vi "LtaGetModuleProperties.vi"(8 "Error In":errorcluster[](array[cluster]), 9 "Event HandlerCall":bool, 10 "arg":string, 11 "Test.lvclass":refnum<class "Test.lvclass">) -> (0 "Error Out":errorcluster[](array[cluster]), 2 "XmlData":string, 3 "Test.lvclass":refnum<class "Test.lvclass">)   [LabVIEW 2018, in "Test.lvclass"]
uses:
  Test.lvclass
  Test.lvclass/Test.ctl
  FGen/MemberClasses/ArbitraryFunction/TypeDefs/Arbs.ctl
  AcPwr/AcPwrPlugins/ChromaAcLoad/TypeDefs/Device(s)Settings.ctl
  AcPwr/AcPwrPlugins/NHRDCPower/TypeDefs/Device(s)Settings.ctl
  AcPwr/AcPwrPlugins/NHRDCPower/TypeDefs/Modules.ctl
  AcPwr/AcPwrPlugins/PacificPowerSource/TypeDefs/Device(s)Settings.ctl
  AcPwr/AcPwrPlugins/NhRegenGridSim/TypeDefs/Device(s)Settings.ctl
  AcPwr/AcPwrPlugins/NhRegenGridSim/TypeDefs/Modules.ctl
  AcPwr/AcPwrPlugins/NHRDCPower/TypeDefs/MeasurementData.ctl
  AcPwr/AcPwrPlugins/ChromaAcLoad/TypeDefs/MeasurementData.ctl
  AcPwr/AcPwrPlugins/ChromaAcLoad/TypeDefs/Measurements.ctl
  AcPwr/AcPwrPlugins/ChromaAcLoad/TypeDefs/MeasurementType.ctl
  Accessors/Read ModuleIDs.vi
  Accessors/Read ErrorSeverity.vi
  <vilib>/Utility/error.llb/Error Cluster From Error Code.vi
  <vilib>/ErrorRing/Error Ring.xnode
  Sync/SyncPlugins/SyncPluginBase/SyncPluginBase.lvclass
  <userlib>/NIST/NISTErrorLib/NISTErrorLib.lvlib
  LV_TestAutomation/Comms_lib/Comms.lvlib
  FGen/FgenPlugins/FgenPluginBaseClass/FgenPluginsBase.lvclass
  Analysis/AnalysisPlugins/AnalysisPluginBaseClass/AnalysisPluginsBase.lvclass
  FGen/MemberClasses/ArbitraryFunction/ArbitraryFunction.lvclass
  AcPwr/AcPwrPlugins/AcPwrBaseClass/AcPwrBase.lvclass
  AcPwr/AcPwrPlugins/ChromaAcLoad/ChromaAcLoad.lvclass
  AcPwr/AcPwrPlugins/PacificPowerSource/PacificPowerSource.lvclass
  AcPwr/AcPwrPlugins/NhRegenGridSim/NHRGridSim.lvclass
  AcPwr/AcPwrPlugins/NHRDCPower/NHRDCPower.lvclass
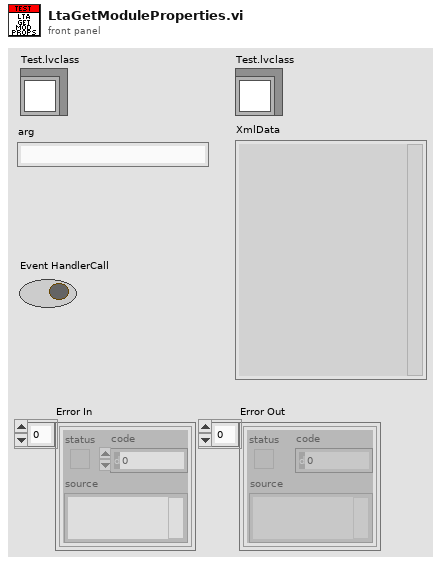
[diagram p1: front panel]
types:
  T1 = typedef "AcPwrPlugins.lvlib/ChromaAcLoad.lvclass/Device(s)Settings.ctl" = cluster{"Configuration Mode":enum16{"Constant Voltage (DC)", "Constant Power (DC)", "Constant Power (AC)", "Constant Current (DC)", "Constant Current (AC)", "Constant Resistance (DC)", "Constant Resistance (AC)", "Rectified Mode (DC)", "Inrush (AC)", "RLC CP (AC)", "RLC (AC)"}, "Phases":cluster{"Handle":string, "Name":string, "Phase Select":i32, "Instrument Options":string, "id query (T)":bool, "reset device (T)":bool, "Load Short Circuited":bool, "Line Synchronization":bool, "Load Current (A/Arms)":dbl, "Load Voltage (V/Vrms)":dbl, "Load Power (W)":dbl, "Load Resistance (Ohms)":dbl, "Load Current Peak Limit (A)":dbl, "Load Current Limit (A/Arms)":dbl, "Load Power Limit (W)":dbl, "Synch Frequency (Hz)":dbl, "Priority":enum16{"CF Only", "PF Only", "Both (CF)", "Both (PF)"}, "Crest Factor":dbl, "Power Factor":dbl, "Slew Rate":cluster{"Rise Slew Rate (A/ms)":i32, "Fall Slew Rate (A/ms)":i32}, "LC/RLC Mode":cluster{"Capacitance (uF)":i32, "Inductance (uH)":i32, "Series Resistance (Ohm)":dbl, "Parallel Resistance (Ohm)":dbl}, "Timing":cluster{"TimingOn":enum16{""}, "Hours":u32, "Minutes":u32, "Seconds":dbl, "CutoffVoltage":dbl}, "Connected":bool}[], "MeasName":string}
  T2 = typedef "AcPwrPlugins.lvlib/PacificPowerSource.lvclass/Device(s)Settings.ctl" = cluster{"MeasName":string, "Modules":cluster{"Handle":string, "Connected":bool, "Clear Device (F)":bool, "btnIdQuery":bool, "btnReset":bool, "Program #":cluster{"Phase B (Degrees)":i32, "Waveform A (1: Sine)":i32, "Voltage Level (Va)":dbl, "Program Number (0)":i32, "Voltage Level (Vb) ":dbl, "Form (3: Three)":u16, "Coupling  (0: Direct)":u16, "Frequency (45Hz)":dbl, "Current Limit (40A)":dbl, "Phase C (Degrees)":i32, "Voltage Level (Vc)":dbl, "Waveform B (1: Sine)":i32, "Waveform C (1: Sine)":i32}[], "Impedance Parameters (off, 0.00)":cluster{"State":bool, "Impedance":dbl}, "Transient Execution (F)":bool, "OutputEnabled":bool, "Source Range":cluster{"Frequency Minimum (45 Hz)":dbl, "Frequency Maximum (1200 Hz)":dbl, "Voltage Maximum (V)":dbl, "Voltage Minimum (V)":dbl, "Range Control (0: Auto)":u16, "Initial Voltage (0V)":u16, "Frequency Range (600Hz)":u16}, "Port Type":enum16{"GPIB", "Serial"}}[]}
  T3 = typedef "AcPwrPlugins.lvlib/NHRGridSim.lvclass/Device(s)Settings.ctl" = cluster{"MeasName":string, "Modules":T4}
  T4 = typedef "AcPwrPlugins.lvlib/NHRGridSim.lvclass/Modules.ctl" = cluster{"Measurement":cluster{"ApertureLength (s)":dbl, "NumberOfSamples":u32}, "Ranges":cluster{"Irange (A)":dbl, "Vrange (V)":dbl}, "Mode":u8, "TransformerRatio":dbl, "Handle":string, "FreqOut (Hz)":dbl, "Connected":bool, "btnIdQuery":bool, "btnReset":bool, "Initialize Timeout ( ms)":u32, "Phase (0: All)":i32, "Grid (0: Normal)":i32, "WatchDog":cluster{"Enable WatchDog":bool, "Robust WatchDog":bool, "Watchdog Interval (s)":dbl}, "Safety Limits":cluster{"Min Voltage (V)":dbl, "Min Voltage Time (s)":dbl, "Max Voltage (V)":dbl, "MaxVoltage Time (s)":dbl, "Max Source Amps (A)":dbl, "Max Source Amps Time (s)":dbl, "Max Sink Amps (A)":dbl, "Max Sink Amps Time (s)":dbl, "Max Source Power (W)":dbl, "Max Source Power Time (s)":dbl, "Max Sink Power (W)":dbl, "Max Sink Power Time (s)":dbl, "Peak Voltage (V)":dbl, "Peak Voltage Enable":bool, "Peak Amps (A)":dbl, "Peak Amps Enable":bool}, "Phases":cluster{"Pout (W)":dbl, "Iout (A)":dbl, "PhaseAngle":dbl, "Vout (V)":dbl, "Phase Name":string}[], "Regulation Gain":dbl, "ChangeOntheFly":bool}[]
  T5 = typedef "AcPwrPlugins.lvlib/ChromaAcLoad.lvclass/MeasurementData.ctl" = cluster{"Time Stamp":timestamp, "Measurements":T6}
  T6 = typedef "AcPwrPlugins.lvlib/ChromaAcLoad.lvclass/Measurements.ctl" = cluster{"Handle":string, "Name":string, "Enabled":bool, "Measurement Value":dbl, "Hold Peak Current Measurement":bool, "btnMeasFetch":bool, "ProtectionStatusString":string, "Measurement Type":T7}[]
  T7 = typedef "AcPwrPlugins.lvlib/ChromaAcLoad.lvclass/MeasurementType.ctl" = enum16{"Voltage (Vrms or V)", "Current (Arms or A)", "Power (W)", "Peak Voltage (V)", "Peak Current (A)", "Peak Power (W)", "Frequency (Hz)", "Resistance (Ohms)", "Voltage Overshoot (V)", "Positive Peak Current (A)", "Voltage Undershoot (V)", "Negative Peak Current (A)", "Apparent Power (VA)", "Reacitive Power (VAR)", "Voltage THD", "Power Factor", "Current's Crest Factor"}
  T8 = typedef "Test.lvclass/SyncEventReg.ctl" = refnum<event-registration>
  T9 = typedef "Test.lvclass/FGenEventReg.ctl" = refnum<event-registration>
  T10 = typedef "Functions.lvlib/ArbitraryFunction.lvclass/Arbs.ctl" = cluster{"Handle":string, "Size":i32, "Gain":dbl, "Offset":dbl}
  T11 = typedef "Test.lvclass/AcPwrEventReg.ctl" = refnum<event-registration>
  T12 = typedef "AcPwrPlugins.lvlib/NHRDCPower.lvclass/Device(s)Settings.ctl" = cluster{"MeasName":string, "Modules":T13}
  T13 = typedef "AcPwrPlugins.lvlib/NHRDCPower.lvclass/Modules.ctl" = cluster{"Handle":string, "Name":string, "id query (Yes)":bool, "reset device (Yes)":bool, "Connected":bool, "Initial Battery Detect Voltage (0)":dbl, "SafetySettings":cluster{"SetWatchDog?":bool, "Voltage (V)":dbl, "Current (A)":dbl, "Power (W)":dbl, "Voltage Delay (s)":dbl, "Current Delay (s)":dbl, "Power Delay (s)":dbl}, "Options String":string, "Aperture Time (s)":dbl, "operating state (Off)":i32, "OutputSettings":cluster{"Voltage (V)":dbl, "Current (A)":dbl, "Resistance (Ohms)":dbl, "Power (W)":dbl, "Enable Voltage":bool, "Enable Current":bool, "Enable Resistance":bool, "Enable Power":bool, "Macro After Step Delay  (s)":dbl, "Wait Value (V, A, W)":dbl, "Enable Wait":bool, "Wait on Value":i32}[], "SlewRate":cluster{"Set Voltage Rate V/S":dbl, "Set Current Rate A/S":dbl, "Set Resistance Rate R/S":dbl, "Set Power Rate W/S":dbl}, "Macro":cluster{"Save Macro?":bool, "Load Macro From File?":bool, "Run Macro Continuously?":bool, "Use Macros?":bool, "Load Macro File Path":string, "Save Macro File Path":string}, "Regulation Gain (1=100%)":dbl, "UpdatingOntheFly":bool}[]
  T14 = typedef "AcPwrPlugins.lvlib/NHRDCPower.lvclass/MeasurementData.ctl" = cluster{"Handle":string, "Measurement Type":enum16{"Power", "Current", "Voltage"}, "Waveform":waveform(sgl)}
  T15 = typedef "Test.lvclass/AnalysisEventReg.ctl" = refnum<event-registration>
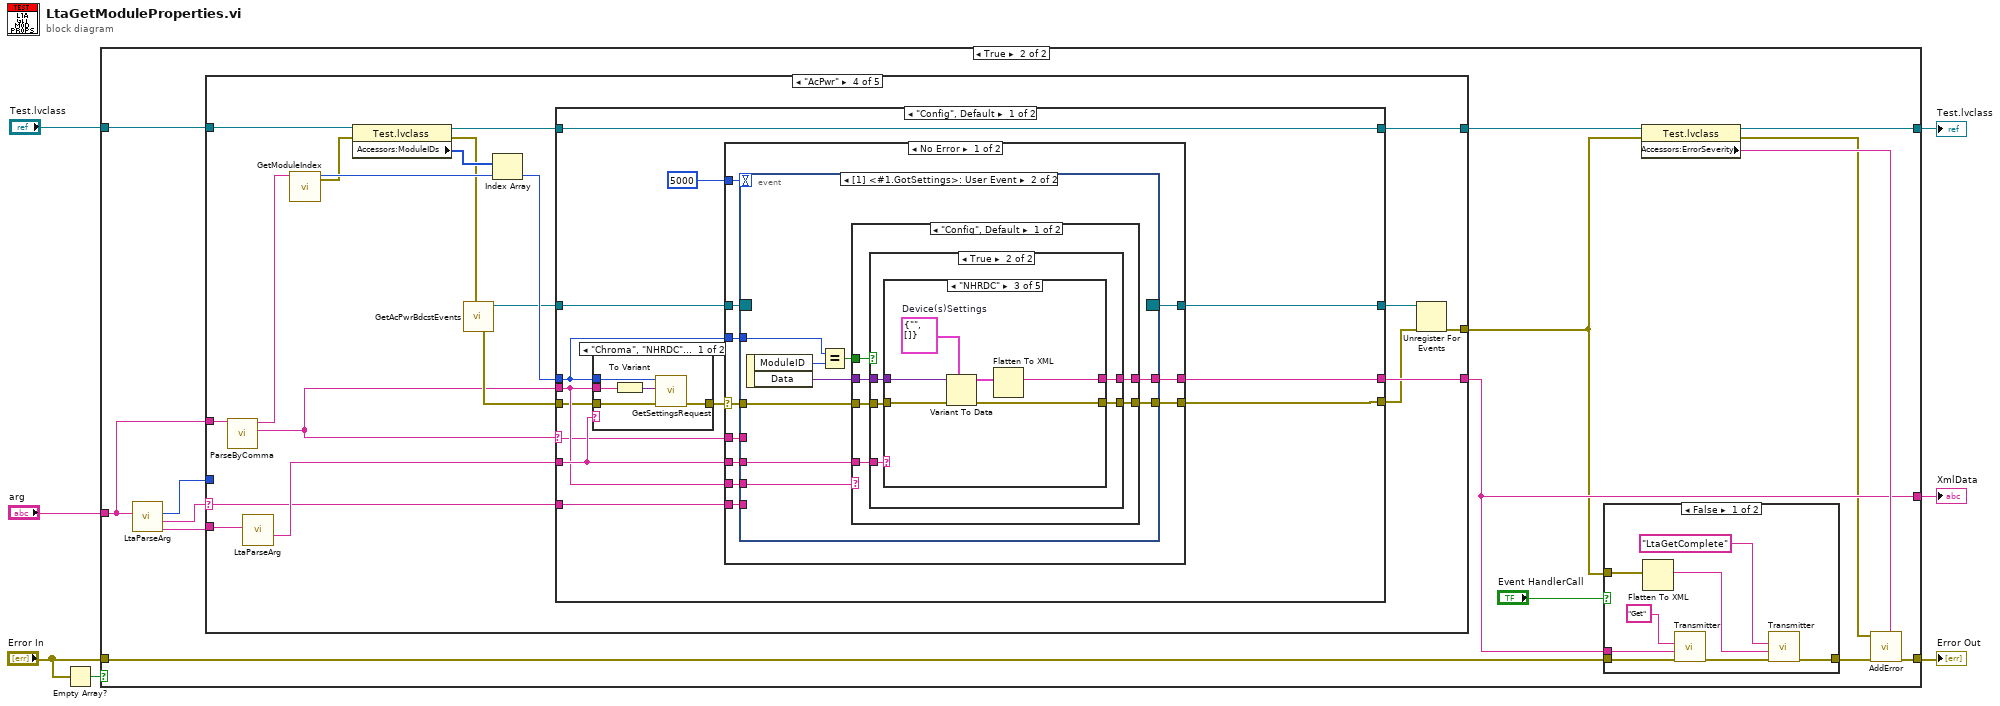
[diagram p0: block diagram]
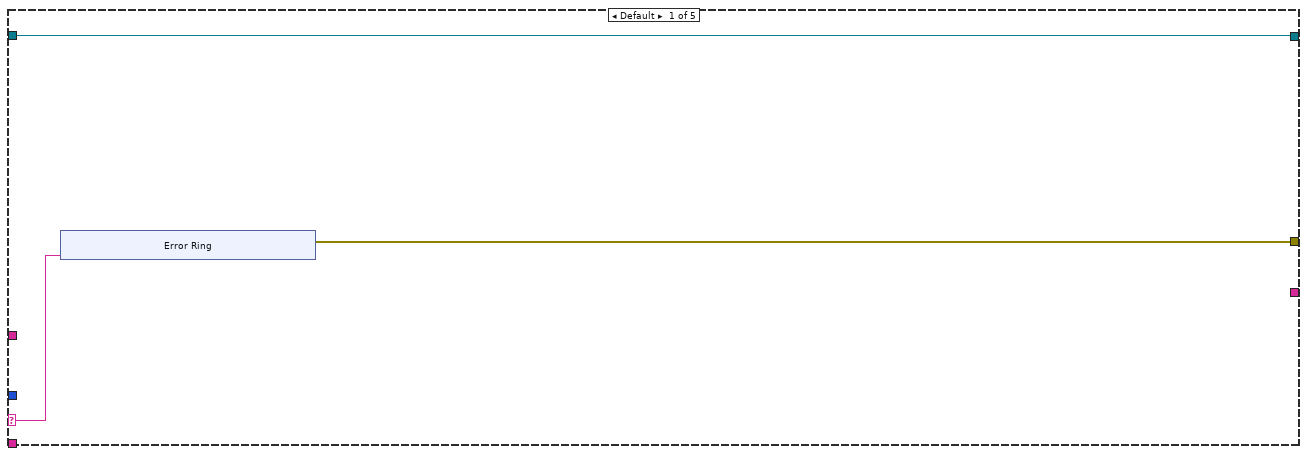
[diagram p4: hidden frame]
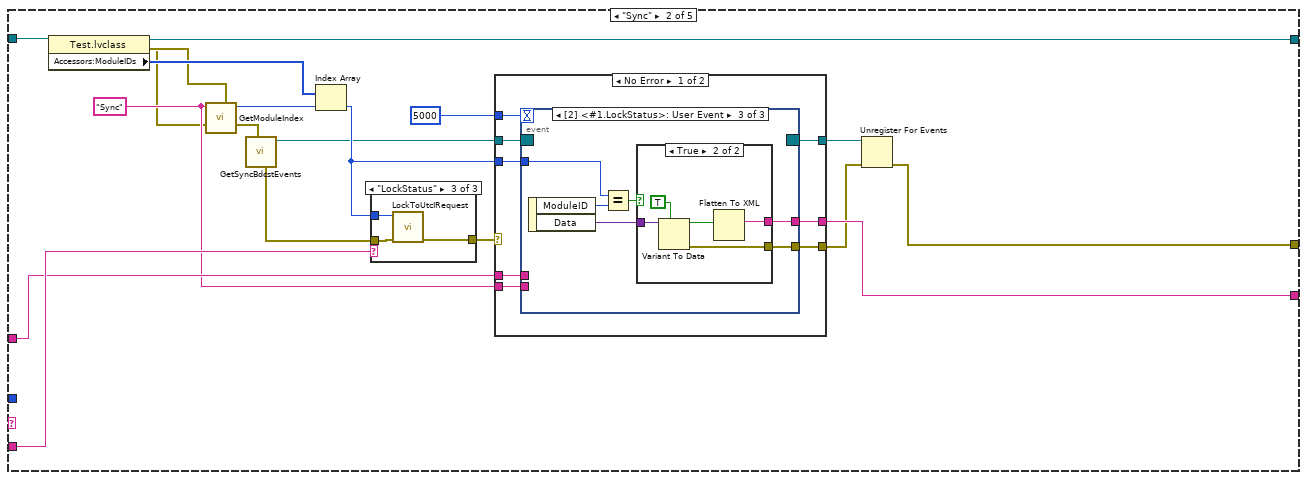
[diagram p5: hidden frame]
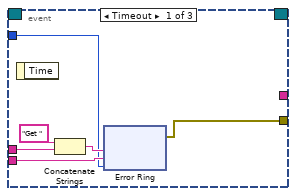
[diagram p6: hidden frame]
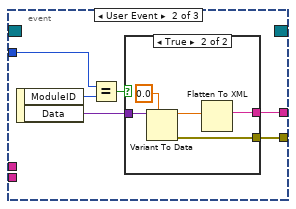
[diagram p7: hidden frame]
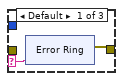
[diagram p11: hidden frame]
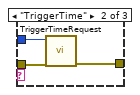
[diagram p12: hidden frame]
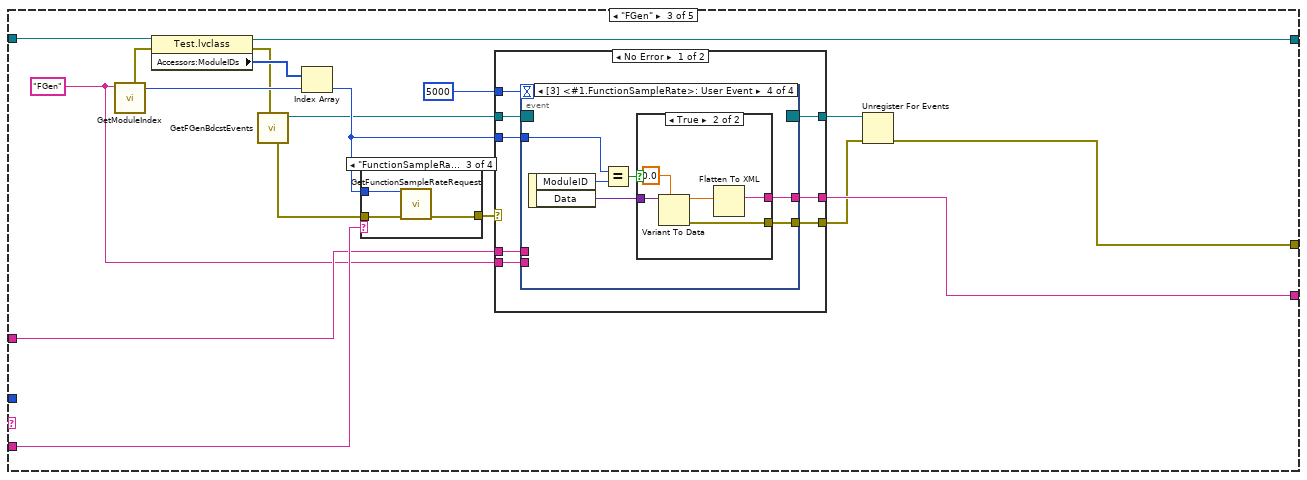
[diagram p13: hidden frame]
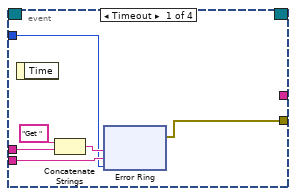
[diagram p14: hidden frame]
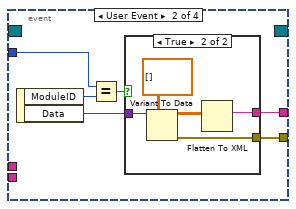
[diagram p15: hidden frame]
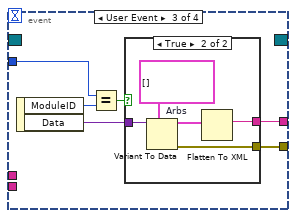
[diagram p17: hidden frame]
diagram:
  n1 = Empty Array?(array="Error In") -> (empty?=w7:bool)
  n2 = case shown="True" w7 {
    tunnel: [w8 w13] -> w6
    tunnel: [w9 w17] -> w4
    tunnel: "Test.lvclass" -> [w9 w20]
    tunnel: "arg" -> [_ w21]
    tunnel: [_ w16] -> w2
    tunnel: "Error In" -> [w8 w14]
    frame False {
    }
    frame True {
      n3 = call "LtaParseArg.vi"("Arg In"=w21) -> ("ArgRemaining"=w23:string, "Arg 1"=w24:string, "Arg1Num"=w22:i32)  [unwired: 8 in]
      n4 = case shown="\"AcPwr\"" w24 {
        selector: w24 -> [w36 _ _ w233 _]
        tunnel: w23 -> [_ w58 w138 w235 w479]
        tunnel: w22 -> [_ _ _ _ _]
        tunnel: w21 -> [_ w55 w134 w231 w474]
        tunnel: [_ w51 w131 w237 w471] -> w16
        tunnel: [w35 w50 w130 w232 w470] -> w12
        tunnel: w20 -> [w34 w49 w129 w236 w480]
        tunnel: [w34 w48 w128 w219 w467] -> w19
        frame Default {
          n5 = xnode "Error Ring"("parameter 0"=w36) -> ("error out"=w35:errorcluster)
        }
        frame "Sync" {
          w54 = "Sync" ("ModuleType")
          n6 = call "GetModuleIndex.vi"("ModuleType"=w54) -> ("ModuleIndex"=w61:i32, "Error"=w59:errorcluster)  [unwired: 9 in]
          n7 = property class="Test.lvclass"(reference=w49, error in=w59) -> (reference out=w48:refnum<class "Test.lvclass">, error out=w44:errorcluster, "Accessors:ModuleIDs"=w60:i32[])
          n8 = call "GetSyncBdcstEvents.vi"("error in (no error)"=w44) -> ("Event Registration Refnum"=w52:T8, "error out"=w45:errorcluster)  [unwired: 9 in]
          n9 = Index Array(array=w60, index=w61) -> (element=w53:i32)
          n10 = case shown="\"LockStatus\"" w58 {
            selector: w58 -> [w110 _ _]
            tunnel: [w109 w118 w121] -> w57
            tunnel: w53 -> [_ w119 w122]
            tunnel: w45 -> [_ w120 w123]
            frame Default {
              n11 = xnode "Error Ring"("parameter 0"=w110) -> ("error out"=w109:errorcluster)
            }
            frame "TriggerTime" {
              n12 = call "TriggerTimeRequest.vi"("error in (no error)"=w120, "ModuleID"=w119) -> ("error out"=w118:errorcluster)  [unwired: 9 in]
            }
            frame "LockStatus" {
              n13 = call "LockToUtcIRequest.vi"("error in (no error)"=w123, "ModuleID"=w122) -> ("error out"=w121:errorcluster)  [unwired: 9 in]
            }
          }
          n14 = case shown="No Error" w57 {
            selector: w57 -> [_ w108]
            tunnel: 5000 -> [w69 _]
            tunnel: w55 -> [w68 _]
            tunnel: w54 -> [w67 _]
            tunnel: w53 -> [w66 _]
            tunnel: w52 -> [w65 w107]
            tunnel: [w64 w107] -> w47
            tunnel: [w63 _] -> w51
            tunnel: [w62 w108] -> w46
            frame No Error {
              n15 = event shown="[2] <#1.LockStatus>: User Event" {
                selector: w65 -> [_ _ _]
                dyn-events: [_ _ _] -> w64
                timeout: w69 -> [_ _ _]
                tunnel: w68 -> [w74 _ _]
                tunnel: w67 -> [w72 _ _]
                tunnel: w66 -> [w71 w89 w100]
                tunnel: [_ w86 w97] -> w63
                tunnel: [w70 w85 w96] -> w62
                event Timeout {
                  n16 = event-data() -> ()  [unwired: 1 in, 1 out]
                  n17 = Concatenate Strings("Get " ("string"), w74) -> (w75:string)
                  n18 = xnode "Error Ring"("parameter 0"=w75, "parameter 1"=w72, "parameter 2"=w71) -> ("error out"=w70:errorcluster)
                }
                event User Event {
                  n19 = event-data() -> ("ModuleID"=w90:i32, "Data"=w87:variant)  [unwired: 1 in]
                  n20 = Equal?(x=w89, y=w90) -> (x = y?=w88:bool)
                  n21 = case shown="True" w88 {
                    tunnel: w87 -> [_ w95]
                    tunnel: [_ w93] -> w85
                    tunnel: [_ w91] -> w86
                    frame False {
                    }
                    frame True {
                      n22 = Variant To Data(type=0.0, Variant=w95) -> (data=w92:dbl, error out=w93:errorcluster)  [unwired: 1 in]
                      n23 = Flatten To XML(anything=w92) -> (xml string=w91:string)
                    }
                  }
                }
                event User Event {
                  n24 = event-data() -> ("ModuleID"=w101:i32, "Data"=w98:variant)  [unwired: 1 in]
                  n25 = Equal?(x=w100, y=w101) -> (x = y?=w99:bool)
                  n26 = case shown="True" w99 {
                    tunnel: w98 -> [_ w106]
                    tunnel: [_ w104] -> w96
                    tunnel: [_ w102] -> w97
                    frame False {
                    }
                    frame True {
                      n27 = Variant To Data(type=TRUE, Variant=w106) -> (data=w103:bool, error out=w104:errorcluster)  [unwired: 1 in]
                      n28 = Flatten To XML(anything=w103) -> (xml string=w102:string)
                    }
                  }
                }
              }
            }
            frame Error {
            }
          }
          n29 = Unregister For Events(event registration refnum=w47, error in=w46) -> (error out=w50:errorcluster)
        }
        frame "FGen" {
          w133 = "FGen" ("ModuleType")
          n30 = call "GetModuleIndex.vi"("ModuleType"=w133) -> ("ModuleIndex"=w141:i32, "Error"=w139:errorcluster)  [unwired: 9 in]
          n31 = property class="Test.lvclass"(reference=w129, error in=w139) -> (reference out=w128:refnum<class "Test.lvclass">, error out=w137:errorcluster, "Accessors:ModuleIDs"=w140:i32[])
          n32 = call "GetFGenBdcstEvents.vi"("error in (no error)"=w137) -> ("Event Registration Refnum"=w125:T9, "error out"=w124:errorcluster)  [unwired: 9 in]
          n33 = Index Array(array=w140, index=w141) -> (element=w132:i32)
          n34 = case shown="\"FunctionSampleRate\"" w138 {
            selector: w138 -> [_ _ _ w210]
            tunnel: [w200 w203 w206 w209] -> w136
            tunnel: w132 -> [w201 w204 w207 _]
            tunnel: w124 -> [w202 w205 w208 _]
            frame "FunctionParams" {
              n35 = call "GetFunctionParamsRequest.vi"("error in (no error)"=w202, "ModuleID"=w201) -> ("error out"=w200:errorcluster)  [unwired: 9 in]
            }
            frame "FunctionArbs" {
              n36 = call "GetFunctionArbsRequest.vi"("error in (no error)"=w205, "ModuleID"=w204) -> ("error out"=w203:errorcluster)  [unwired: 9 in]
            }
            frame "FunctionSampleRate" {
              n37 = call "GetFunctionSampleRateRequest.vi"("error in (no error)"=w208, "ModuleID"=w207) -> ("error out"=w206:errorcluster)  [unwired: 9 in]
            }
            frame Default {
              n38 = xnode "Error Ring"("parameter 0"=w210) -> ("error out"=w209:errorcluster)
            }
          }
          n39 = case shown="No Error" w136 {
            selector: w136 -> [_ w199]
            tunnel: 5000 -> [w149 _]
            tunnel: w134 -> [w148 _]
            tunnel: w133 -> [w147 _]
            tunnel: w132 -> [w146 _]
            tunnel: w125 -> [w145 w198]
            tunnel: [w144 w198] -> w127
            tunnel: [w143 _] -> w131
            tunnel: [w142 w199] -> w126
            frame No Error {
              n40 = event shown="[3] <#1.FunctionSampleRate>: User Event" {
                selector: w145 -> [_ _ _ _]
                dyn-events: [_ _ _ _] -> w144
                timeout: w149 -> [_ _ _ _]
                tunnel: w148 -> [w154 _ _ _]
                tunnel: w147 -> [w152 _ _ _]
                tunnel: w146 -> [w151 w169 w180 w191]
                tunnel: [_ w166 w177 w188] -> w143
                tunnel: [w150 w165 w176 w187] -> w142
                event Timeout {
                  n41 = event-data() -> ()  [unwired: 1 in, 1 out]
                  n42 = Concatenate Strings("Get " ("string"), w154) -> (w155:string)
                  n43 = xnode "Error Ring"("parameter 0"=w155, "parameter 1"=w152, "parameter 2"=w151) -> ("error out"=w150:errorcluster)
                }
                event User Event {
                  n44 = event-data() -> ("ModuleID"=w170:i32, "Data"=w167:variant)  [unwired: 1 in]
                  n45 = Equal?(x=w169, y=w170) -> (x = y?=w168:bool)
                  n46 = case shown="True" w168 {
                    tunnel: w167 -> [_ w175]
                    tunnel: [_ w174] -> w165
                    tunnel: [_ w172] -> w166
                    frame False {
                    }
                    frame True {
                      n47 = Variant To Data(type=dbl[][] [], Variant=w175) -> (data=w173:dbl[][], error out=w174:errorcluster)  [unwired: 1 in]
                      n48 = Flatten To XML(anything=w173) -> (xml string=w172:string)
                    }
                  }
                }
                event User Event {
                  n49 = event-data() -> ("ModuleID"=w181:i32, "Data"=w178:variant)  [unwired: 1 in]
                  n50 = Equal?(x=w180, y=w181) -> (x = y?=w179:bool)
                  n51 = case shown="True" w179 {
                    tunnel: w178 -> [_ w186]
                    tunnel: [_ w185] -> w176
                    tunnel: [_ w183] -> w177
                    frame False {
                    }
                    frame True {
                      w182 = T10[] []  # Arbs
                      n52 = Variant To Data(type=w182, Variant=w186) -> (data=w184:T10[], error out=w185:errorcluster)  [unwired: 1 in]
                      n53 = Flatten To XML(anything=w184) -> (xml string=w183:string)
                    }
                  }
                }
                event User Event {
                  n54 = event-data() -> ("ModuleID"=w192:i32, "Data"=w189:variant)  [unwired: 1 in]
                  n55 = Equal?(x=w191, y=w192) -> (x = y?=w190:bool)
                  n56 = case shown="True" w190 {
                    tunnel: w189 -> [_ w197]
                    tunnel: [_ w196] -> w187
                    tunnel: [_ w194] -> w188
                    frame False {
                    }
                    frame True {
                      n57 = Variant To Data(type=0.0, Variant=w197) -> (data=w195:dbl, error out=w196:errorcluster)  [unwired: 1 in]
                      n58 = Flatten To XML(anything=w195) -> (xml string=w194:string)
                    }
                  }
                }
              }
            }
            frame Error {
            }
          }
          n59 = Unregister For Events(event registration refnum=w127, error in=w126) -> (error out=w130:errorcluster)
        }
        frame "AcPwr" {
          n60 = call "ParseByComma.vi"("String"=w231) -> ("SecondParseValue"=w218:string, "FirstParseValue"=w230:string)  [unwired: 8 in, 1 out]
          n61 = call "LtaParseArg.vi"("Arg In"=w235) -> ("Arg 1"=w234:string)  [unwired: 8 in, 2 out]
          n62 = call "GetModuleIndex.vi"("ModuleType"=w230) -> ("ModuleIndex"=w229:i32, "Error"=w227:errorcluster)  [unwired: 9 in]
          n63 = property class="Test.lvclass"(reference=w236, error in=w227) -> (reference out=w220:refnum<class "Test.lvclass">, error out=w223:errorcluster, "Accessors:ModuleIDs"=w228:i32[])
          n64 = call "GetAcPwrBdcstEvents.vi"("error in (no error)"=w223) -> ("Event Registration Refnum"=w221:T11, "error out"=w222:errorcluster)  [unwired: 9 in]
          n65 = Index Array(array=w228, index=w229) -> (element=w226:i32)
          n66 = case shown="\"Config\", Default" w218 {
            selector: w218 -> [w246 w366]
            tunnel: [w250 w370] -> w237
            tunnel: w234 -> [w249 w369]
            tunnel: w233 -> [w248 w368]
            tunnel: w218 -> [w247 w367]
            tunnel: w226 -> [w244 w364]
            tunnel: [w243 w363] -> w225
            tunnel: [w242 w362] -> w224
            tunnel: w222 -> [w241 w359]
            tunnel: w221 -> [w240 w361]
            tunnel: w220 -> [w238 w360]
            tunnel: [w238 w360] -> w219
            frame "Config", Default {
              n67 = case shown="\"Chroma\", \"NHRDC\", \"NHRRegen\", \"PPS\"" w249 {
                selector: w249 -> [_ w351]
                tunnel: [w348 w350] -> w239
                tunnel: w244 -> [w347 _]
                tunnel: w241 -> [w349 _]
                tunnel: w247 -> [w345 _]
                frame "Chroma", "NHRDC", "NHRRegen", "PPS" {
                  n68 = To Variant(anything=w345) -> (Variant=w346:variant)
                  n69 = call "GetSettingsRequest.vi"("Error In"=w349, "SettingsToGet"=w346, "ModuleID"=w347) -> ("Error Out"=w348:errorcluster)  [unwired: 8 in]
                }
                frame Default {
                  n70 = xnode "Error Ring"("parameter 0"=w351) -> ("error out"=w350:errorcluster)
                }
              }
              n71 = case shown="No Error" w239 {
                selector: w239 -> [w253 w344]
                tunnel: 5000 -> [w261 _]
                tunnel: w246 -> [w260 _]
                tunnel: w248 -> [w259 _]
                tunnel: w244 -> [w258 _]
                tunnel: w240 -> [w257 w343]
                tunnel: [w256 w343] -> w243
                tunnel: [w255 _] -> w250
                tunnel: [w254 w344] -> w242
                tunnel: w249 -> [w252 _]
                tunnel: w247 -> [w251 _]
                frame No Error {
                  n72 = event shown="[1] <#1.GotSettings>: User Event" {
                    selector: w257 -> [_ _]
                    dyn-events: [_ _] -> w256
                    timeout: w261 -> [_ _]
                    tunnel: w260 -> [w266 _]
                    tunnel: w259 -> [w264 _]
                    tunnel: w258 -> [w263 w284]
                    tunnel: [_ w281] -> w255
                    tunnel: [w262 w280] -> w254
                    tunnel: w253 -> [_ w279]
                    tunnel: w252 -> [_ w278]
                    tunnel: w251 -> [_ w277]
                    event Timeout {
                      n73 = event-data() -> ()  [unwired: 1 in, 1 out]
                      n74 = Concatenate Strings("Get " ("string"), w266) -> (w267:string)
                      n75 = xnode "Error Ring"("parameter 0"=w267, "parameter 1"=w264, "parameter 2"=w263) -> ("error out"=w262:errorcluster)
                    }
                    event User Event {
                      n76 = event-data() -> ("ModuleID"=w285:i32, "Data"=w282:variant)  [unwired: 1 in]
                      n77 = Equal?(x=w284, y=w285) -> (x = y?=w283:bool)
                      n78 = case shown="\"Config\", Default" w277 {
                        tunnel: w283 -> [w291 w331]
                        tunnel: w282 -> [w290 w335]
                        tunnel: [w289 w333] -> w281
                        tunnel: [w288 w334] -> w280
                        tunnel: w279 -> [w287 w332]
                        tunnel: w278 -> [w286 _]
                        frame "Config", Default {
                          n79 = case shown="True" w291 {
                            tunnel: w290 -> [_ w297]
                            tunnel: [w292 w294] -> w288
                            tunnel: [_ w295] -> w289
                            tunnel: w287 -> [w292 w296]
                            tunnel: w286 -> [_ w293]
                            frame False {
                            }
                            frame True {
                              n80 = case shown="\"NHRDC\"" w293 {
                                selector: w293 -> [w299 _ _ _ _]
                                tunnel: [_ w311 w314 w322 w330] -> w295
                                tunnel: [w298 w310 w315 w323 w329] -> w294
                                tunnel: w296 -> [_ w309 w316 w321 w328]
                                tunnel: w297 -> [_ w308 w317 w320 w327]
                                frame Default {
                                n81 = xnode "Error Ring"("parameter 0"=w299) -> ("error out"=w298:errorcluster)
                                }
                                frame "Chroma" {
                                n82 = Variant To Data(error in=w309, type=T1 {"Configuration Mode"=enum."Constant Voltage (DC)", "Phases"=[], "MeasName"=""} ("Chroma"), Variant=w308) -> (data=w312:T1, error out=w310:errorcluster)
                                n83 = Flatten To XML(anything=w312) -> (xml string=w311:string)
                                }
                                frame "NHRDC" {
                                w313 = T12 {"MeasName"="", "Modules"=[]}  # Device(s)Settings
                                n84 = Variant To Data(error in=w316, type=w313, Variant=w317) -> (data=w318:T12, error out=w315:errorcluster)
                                n85 = Flatten To XML(anything=w318) -> (xml string=w314:string)
                                }
                                frame "PPS" {
                                n86 = Variant To Data(error in=w321, type=T2 {"MeasName"="", "Modules"=[]} ("Device(s)Settings"), Variant=w320) -> (data=w324:T2, error out=w323:errorcluster)
                                n87 = Flatten To XML(anything=w324) -> (xml string=w322:string)
                                }
                                frame "NHRRGS" {
                                n88 = Variant To Data(error in=w328, type=T3 {"MeasName"="", "Modules"=[]} ("Device(s)Settings"), Variant=w327) -> (data=w326:T3, error out=w329:errorcluster)
                                n89 = Flatten To XML(anything=w326) -> (xml string=w330:string)
                                }
                              }
                            }
                          }
                        }
                        frame "MRT" {
                          n90 = case shown="True" w331 {
                            tunnel: w335 -> [_ w342]
                            tunnel: [w336 w339] -> w334
                            tunnel: [_ w340] -> w333
                            tunnel: w332 -> [w336 w341]
                            frame False {
                            }
                            frame True {
                              n91 = Variant To Data(error in=w341, type=u32 0, Variant=w342) -> (data=w338:u32, error out=w339:errorcluster)
                              n92 = Flatten To XML(anything=w338) -> (xml string=w340:string)
                            }
                          }
                        }
                      }
                    }
                  }
                }
                frame Error {
                }
              }
            }
            frame "Meas" {
              n93 = case shown="No Error" w359 {
                selector: w359 -> [w374 w465]
                tunnel: 5000 -> [w381 _]
                tunnel: w366 -> [w380 _]
                tunnel: w368 -> [w379 _]
                tunnel: w364 -> [w378 _]
                tunnel: w361 -> [w377 w464]
                tunnel: [w376 w464] -> w363
                tunnel: [w375 _] -> w370
                tunnel: [w371 w465] -> w362
                tunnel: w369 -> [w373 _]
                tunnel: w367 -> [w372 _]
                frame No Error {
                  n94 = while {
                    tunnel: w381 -> [w394]
                    tunnel: w379 -> [w392]
                    tunnel: w378 -> [w391]
                    tunnel: w373 -> [w386]
                    tunnel: w372 -> [w385]
                    shift-right: [w388] -> w375
                    shift-left: w380 -> [w393]
                    shift-right: [w389] -> w376
                    shift-left: w377 -> [w390]
                    shift-right: [w384] -> w371
                    shift-left: w374 -> [w387]
                    stop <- w382 stop-if-true
                    n95 = event shown="[1] <#1.Measurements>: User Event" {
                      selector: w390 -> [_ _]
                      dyn-events: [_ _] -> w389
                      timeout: w394 -> [_ _]
                      tunnel: w393 -> [w400 _]
                      tunnel: w392 -> [w398 _]
                      tunnel: w391 -> [w397 w418]
                      tunnel: [_ w416] -> w388
                      tunnel: [w396 w417] -> w384
                      tunnel: w387 -> [_ w413]
                      tunnel: w386 -> [_ w412]
                      tunnel: w385 -> [_ _]
                      tunnel: [FALSE w411] -> w383
                      event Timeout {
                        n96 = event-data() -> ()  [unwired: 1 in, 1 out]
                        n97 = Concatenate Strings("Get " ("string"), w400) -> (w401:string)
                        n98 = xnode "Error Ring"("parameter 0"=w401, "parameter 1"=w398, "parameter 2"=w397) -> ("error out"=w396:errorcluster)
                      }
                      event User Event {
                        n99 = event-data() -> ("Data"=w415:variant, "ModuleID"=w419:i32)  [unwired: 1 in]
                        n100 = Equal?(x=w419, y=w418) -> (x = y?=w414:bool)
                        n101 = case shown="True" w414 {
                          selector: w414 -> [_ w422]
                          tunnel: w415 -> [_ w427]
                          tunnel: [w420 w424] -> w417
                          tunnel: [_ w425] -> w416
                          tunnel: w413 -> [w420 w426]
                          tunnel: w412 -> [_ w423]
                          tunnel: [_ w421] -> w411
                          frame False {
                          }
                          frame True {
                            n102 = case shown="\"NHRDC\"" w423 {
                              selector: w423 -> [w429 _ _ _ _]
                              tunnel: [_ w443 w451 w455 w463] -> w425
                              tunnel: [w428 w439 w447 w456 w462] -> w424
                              tunnel: w426 -> [_ w442 w450 w454 w461]
                              tunnel: w427 -> [_ w441 w449 w453 w460]
                              tunnel: w422 -> [_ w440 w448 _ _]
                              tunnel: [_ w440 w448 _ _] -> w421
                              frame Default {
                                n103 = xnode "Error Ring"("parameter 0"=w429) -> ("error out"=w428:errorcluster)
                              }
                              frame "NHRDC" {
                                w438 = T14 {"Handle"="", "Measurement Type"=enum."Power", "Waveform"={"t0"=timestamp(0 s since 1904-01-01), "dt"=1.0, "Y"=[]}}  # Measurement Cluster
                                n104 = Variant To Data(error in=w442, type=w438, Variant=w441) -> (data=w437:T14, error out=w439:errorcluster)
                                n105 = Flatten To XML(anything=w437) -> (xml string=w443:string)
                              }
                              frame "Chroma" {
                                n106 = Variant To Data(error in=w450, type=T5 {"Time Stamp"=timestamp(0 s since 1904-01-01), "Measurements"=[]} ("MeasurementData"), Variant=w449) -> (data=w446:T5, error out=w447:errorcluster)
                                n107 = Unbundle By Name(w446) -> ("Measurements"=w445:T6)
                                n108 = Flatten To XML(anything=w445) -> (xml string=w451:string)
                              }
                              frame "PPS" {
                                n109 = Variant To Data(error in=w454, type=T2 {"MeasName"="", "Modules"=[]} ("Device(s)Settings"), Variant=w453) -> (data=w457:T2, error out=w456:errorcluster)
                                n110 = Flatten To XML(anything=w457) -> (xml string=w455:string)
                              }
                              frame "NHRRGS" {
                                n111 = Variant To Data(error in=w461, type=T3 {"MeasName"="", "Modules"=[]} ("Device(s)Settings"), Variant=w460) -> (data=w459:T3, error out=w462:errorcluster)
                                n112 = Flatten To XML(anything=w459) -> (xml string=w463:string)
                              }
                            }
                          }
                        }
                      }
                    }
                    n113 = Or(x=w384, y=w383) -> (x .or. y?=w382:bool)
                  }
                }
                frame Error {
                }
              }
            }
          }
          n114 = Unregister For Events(event registration refnum=w225, error in=w224) -> (error out=w232:errorcluster)
        }
        frame "Analysis" {
          w473 = "Analysis" ("ModuleType")
          n115 = call "GetModuleIndex.vi"("ModuleType"=w473) -> ("ModuleIndex"=w483:i32, "Error"=w481:errorcluster)  [unwired: 9 in]
          n116 = property class="Test.lvclass"(reference=w480, error in=w481) -> (reference out=w467:refnum<class "Test.lvclass">, error out=w478:errorcluster, "Accessors:ModuleIDs"=w482:i32[])
          n117 = call "GetAnalysisBdcstEvents.vi"("error in (no error)"=w478) -> ("Event Registration Refnum"=w476:T15, "error out"=w466:errorcluster)  [unwired: 9 in]
          n118 = Index Array(array=w482, index=w483) -> (element=w472:i32)
          n119 = case shown="\"State\"" w479 {
            selector: w479 -> [_ w526]
            tunnel: [w522 w525] -> w477
            tunnel: w466 -> [w524 _]
            tunnel: w472 -> [w523 _]
            frame "State" {
              n120 = call "GetStateRequest.vi"("error in (no error)"=w524, "ModuleID"=w523) -> ("error out"=w522:errorcluster)  [unwired: 9 in]
            }
            frame Default {
              n121 = xnode "Error Ring"("parameter 0"=w526) -> ("error out"=w525:errorcluster)
            }
          }
          n122 = case shown="No Error" w477 {
            selector: w477 -> [w487 w521]
            tunnel: w476 -> [w492 w520]
            tunnel: 5000 -> [w491 _]
            tunnel: w474 -> [w490 _]
            tunnel: w473 -> [w489 _]
            tunnel: w472 -> [w488 _]
            tunnel: [w486 _] -> w471
            tunnel: [w485 w521] -> w468
            tunnel: [w484 w520] -> w469
            frame No Error {
              n123 = event shown="[1] <#1.State>: User Event" {
                selector: w492 -> [_ _]
                dyn-events: [_ _] -> w484
                timeout: w491 -> [_ _]
                tunnel: w490 -> [w495 _]
                tunnel: w489 -> [w494 _]
                tunnel: w488 -> [w493 w512]
                tunnel: w487 -> [_ w509]
                tunnel: [_ w508] -> w486
                tunnel: [_ w507] -> w485
                event Timeout {
                  n124 = event-data() -> ()  [unwired: 1 in, 1 out]
                  n125 = Concatenate Strings("Get " ("string"), w495) -> (w497:string)
                  n126 = xnode "Error Ring"("parameter 0"=w497, "parameter 1"=w494, "parameter 2"=w493) -> ()  [unwired: 1 out]
                }
                event User Event {
                  n127 = event-data() -> ("ModuleID"=w513:i32, "Data"=w510:variant)  [unwired: 1 in]
                  n128 = Equal?(x=w512, y=w513) -> (x = y?=w511:bool)
                  n129 = case shown="True" w511 {
                    tunnel: w510 -> [_ w518]
                    tunnel: w509 -> [_ w519]
                    tunnel: [_ w515] -> w508
                    tunnel: [_ w514] -> w507
                    frame False {
                    }
                    frame True {
                      n130 = Variant To Data(error in=w519, type="", Variant=w518) -> (data=w516:string, error out=w514:errorcluster)
                      n131 = Flatten To XML(anything=w516) -> (xml string=w515:string)
                    }
                  }
                }
              }
            }
            frame Error {
            }
          }
          n132 = Unregister For Events(event registration refnum=w469, error in=w468) -> (error out=w470:errorcluster)
        }
      }
      n133 = case shown="False" "Event HandlerCall" {
        tunnel: w16 -> [w32 _]
        tunnel: [w29 w33] -> w15
        tunnel: w14 -> [w26 w33]
        tunnel: w12 -> [w25 _]
        frame False {
          n134 = Flatten To XML(anything=w25) -> (xml string=w27:string)
          n135 = call "Transmitter.vi"("ErrorArray"=w26, "XMLData"=w32, "Command"="Get") -> ("ErrorArray"=w30:errorcluster[])  [unwired: 7 in, 1 out]
          n136 = call "Transmitter.vi"("ErrorArray"=w30, "XMLData"=w27, "Command"="LtaGetComplete") -> ("ErrorArray"=w29:errorcluster[])  [unwired: 7 in, 1 out]
        }
        frame True {
        }
      }
      n137 = property class="Test.lvclass"(reference=w19, error in=w12) -> (reference out=w17:refnum<class "Test.lvclass">, error out=w11:errorcluster, "Accessors:ErrorSeverity"=w18:string)
      n138 = call <userlib>:"AddError.vi"("Severity"=w18, "ErrorArray"=w15, "error in (no error)"=w11) -> ("ErrorArray"=w13:errorcluster[])  [unwired: 7 in, 1 out]
    }
  }
  "Test.lvclass" <- w4
  "Error Out" <- w6
  "XmlData" <- w2
